vi "update and log odors.vi"(4 "odor 1 enabled?":bool=TRUE, 7 "global enable":bool, 8 "error in":errorcluster, 9 "t0":u32, 10 "gradient settings":T3={"air settings"={"enabled"=FALSE, "temporal ramp type"=enum."Sine", "period(s)"=120.0, "high limit"=100.0, "low limit"=0.0, "duty cycle (sq wave)"=50.0, "phase shift (deg)"=0.0, "value to output when disabled"=0.0}, "odor1 settings"={"enabled"=FALSE, "temporal ramp type"=enum."Sine", "period(s)"=120.0, "high limit"=100.0, "low limit"=0.0, "duty cycle (sq wave)"=50.0, "phase shift (deg)"=0.0, "value to output when disabled"=0.0}, "odor2 settings"={"enabled"=FALSE, "temporal ramp type"=enum."Sine", "period(s)"=120.0, "high limit"=100.0, "low limit"=0.0, "duty cycle (sq wave)"=50.0, "phase shift (deg)"=0.0, "value to output when disabled"=0.0}, "co2 settings"={"enabled"=FALSE, "temporal ramp type"=enum."Sine", "period(s)"=120.0, "high limit"=100.0, "low limit"=0.0, "duty cycle (sq wave)"=50.0, "phase shift (deg)"=0.0, "value to output when disabled"=0.0}} {"co2 settings"."value to output when disabled" max=100.0; "co2 settings"."low limit" min=0.0 max=1.0 format="%#_6p"; "co2 settings"."high limit" max=100.0; "odor2 settings"."value to output when disabled" max=100.0; "odor2 settings"."low limit" min=0.0 max=1.0 format="%#_6p"; "odor2 settings"."high limit" max=100.0; "odor1 settings"."value to output when disabled" max=100.0; "odor1 settings"."low limit" min=0.0 max=1.0 format="%#_6p"; "odor1 settings"."high limit" max=100.0; "air settings"."value to output when disabled" max=100.0; "air settings"."low limit" min=0.0 max=1.0 format="%#_6p"; "air settings"."high limit" max=100.0}, 11 "daqmx tasks":T4) -> (0 "error out":errorcluster, 2 "flow rates":T1 {"pid reading" format="%0.2f"}, 3 "setpoints":T2)   [LabVIEW 2021]
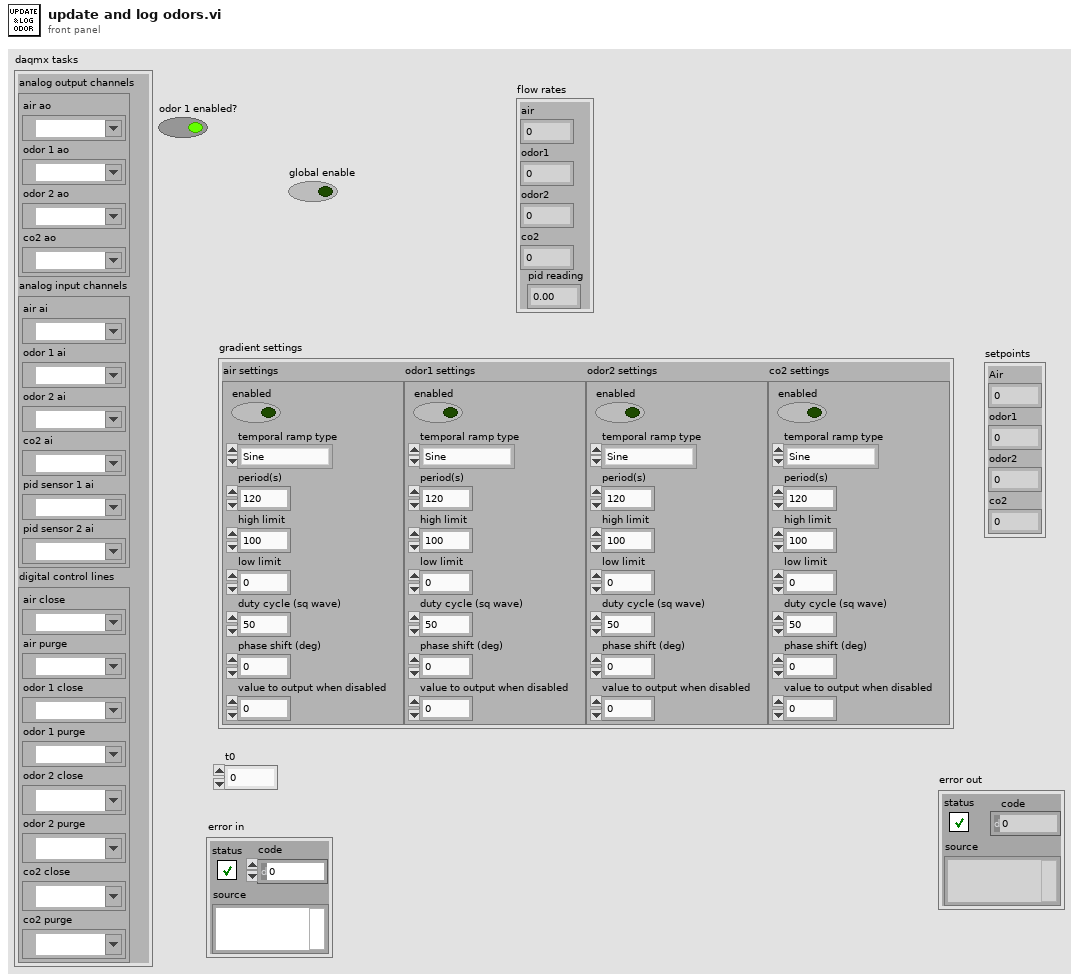
[diagram p1: front panel]
types:
  T1 = cluster{"air":dbl, "odor1":dbl, "odor2":dbl, "co2":dbl, "pid reading":dbl}
  T2 = cluster{"Air ":dbl, "odor1":dbl, "odor2":dbl, "co2":dbl}
  T3 = cluster{"air settings":cluster{"enabled":bool, "temporal ramp type":enum16{"Sine", "Triangle", "Sawtooth", "Square", "Exponential"}, "period(s)":dbl, "high limit":dbl, "low limit":dbl, "duty cycle (sq wave)":dbl, "phase shift (deg)":dbl, "value to output when disabled":dbl}, "odor1 settings":cluster{"enabled":bool, "temporal ramp type":enum16{"Sine", "Triangle", "Sawtooth", "Square", "Exponential"}, "period(s)":dbl, "high limit":dbl, "low limit":dbl, "duty cycle (sq wave)":dbl, "phase shift (deg)":dbl, "value to output when disabled":dbl}, "odor2 settings":cluster{"enabled":bool, "temporal ramp type":enum16{"Sine", "Triangle", "Sawtooth", "Square", "Exponential"}, "period(s)":dbl, "high limit":dbl, "low limit":dbl, "duty cycle (sq wave)":dbl, "phase shift (deg)":dbl, "value to output when disabled":dbl}, "co2 settings":cluster{"enabled":bool, "temporal ramp type":enum16{"Sine", "Triangle", "Sawtooth", "Square", "Exponential"}, "period(s)":dbl, "high limit":dbl, "low limit":dbl, "duty cycle (sq wave)":dbl, "phase shift (deg)":dbl, "value to output when disabled":dbl}}
  T4 = cluster{"analog output channels":cluster{"air ao":refnum<k21>, "odor 1 ao":refnum<k21>, "odor 2 ao":refnum<k21>, "co2 ao":refnum<k21>}, "analog input channels":cluster{"air ai":refnum<k21>, "odor 1 ai":refnum<k21>, "odor 2 ai":refnum<k21>, "co2 ai":refnum<k21>, "pid sensor 1 ai":refnum<k21>, "pid sensor 2 ai":refnum<k21>}, "digital control lines":cluster{"air close":refnum<k21>, "air purge":refnum<k21>, "odor 1 close":refnum<k21>, "odor 1 purge":refnum<k21>, "odor 2 close":refnum<k21>, "odor 2 purge":refnum<k21>, "co2 close":refnum<k21>, "co2 purge":refnum<k21>}}
  T5 = cluster{"enabled":bool, "temporal ramp type":enum16{"Sine", "Triangle", "Sawtooth", "Square", "Exponential"}, "period(s)":dbl, "high limit":dbl, "low limit":dbl, "duty cycle (sq wave)":dbl, "phase shift (deg)":dbl, "value to output when disabled":dbl}[]
  T6 = enum16{"Sine", "Triangle", "Sawtooth", "Square", "Exponential"}
  T7 = cluster{"temporal ramp type":enum16{"Sine", "Triangle", "Sawtooth", "Square", "Exponential"}, "period(s)":dbl, "high limit":dbl, "low limit":dbl, "duty cycle (sq wave)":dbl, "phase shift (deg)":dbl, "value to output when disabled":dbl}
  T8 = cluster{"[0]":dbl, "[1]":dbl, "[2]":dbl, "[3]":dbl}
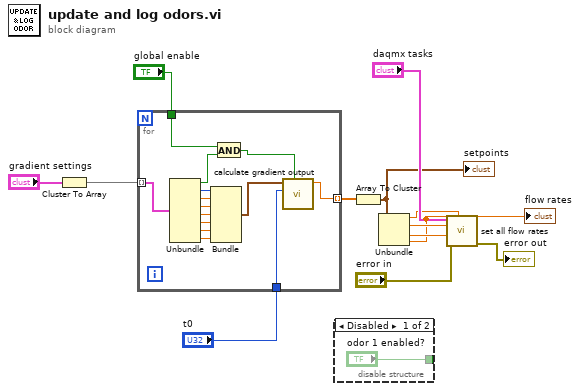
[diagram p0: block diagram]
diagram:
  n1 = Cluster To Array(cluster="gradient settings") -> (array=w11:T5)
  n2 = for {
    tunnel: w11 -> [w27] mode=indexing
    tunnel: "t0" -> [w18]
    tunnel: "global enable" -> [w16]
    tunnel: [w14] -> w8 mode=indexing
    n3 = Unbundle(w27) -> ("enabled"=w17:bool, "temporal ramp type"=w26:T6, "period(s)"=w20:dbl, "high limit"=w21:dbl, "low limit"=w22:dbl, "duty cycle (sq wave)"=w23:dbl, "phase shift (deg)"=w24:dbl, "value to output when disabled"=w25:dbl)
    n4 = Bundle("temporal ramp type"=w26, "period(s)"=w20, "high limit"=w21, "low limit"=w22, "duty cycle (sq wave)"=w23, "phase shift (deg)"=w24, "value to output when disabled"=w25) -> (w19:T7)  [unwired: 1 in]
    n5 = And(x=w16, y=w17) -> (x .and. y?=w15:bool)
    n6 = call "calculate gradient output.vi"("enabled"=w15, "t0"=w18, "gradient parameters"=w19) -> ("value out"=w14:dbl)  [unwired: 8 in]
  }
  n7 = disable-structure shown="Disabled" {
    disable-tunnel: ["odor 1 enabled?" _] -> _
    frame Disabled {
    }
    frame Enabled {
    }
  }
  n8 = Array To Cluster(array=w8) -> (cluster=w7:T8)
  "setpoints" <- w7
  n9 = Unbundle(w7) -> ("[0]"=w6:dbl, "[1]"=w5:dbl, "[2]"=w4:dbl, "[3]"=w1:dbl)
  "flow rates" <- w1
  n10 = call "set all flow rates.vi"("flow rates"=w1, "background air flow rate"=w6, "error in"="error in", "dilution air flow rate"=w4, "odor 1 flow rate"=w5, "LabJack Tasks"="daqmx tasks") -> ("error out"=→"error out":errorcluster)  [unwired: 5 in]
